vi "Shoot Teleop Handler.vi"(11 "Input Velocities":T1) -> ()   [LabVIEW 2025]
uses:
  swerve-template/Type Definitions/Data/Robot Velocities.ctl
  <vilib>/Rock Robotics/WPI/Joystick/XBox Buttons Indexer.ctl
  <vilib>/Rock Robotics/WPI/Joystick/XBox Axes Indexer.ctl
  Hopper/Implementation/Hopper Operations.ctl
  Transfer/Implementation/Transfer Operations.ctl
  Shooter/Implementation/Shooter Operations.ctl
  <vilib>/Rock Robotics/WPI/Utilities/WPI_GetSetVariantRefNum.vi
panel:
  in  "Steal Hood Setpoint":dbl=19.0
  in  "Steal Shot Velocity":dbl=8000.0
  in  "Hoard Hood Setpoint":dbl=19.0
  in  "Hoard Shot Velocity":dbl=4800.0
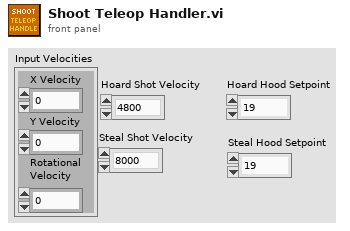
[diagram p1: front panel]
types:
  T1 = typedef "Robot Velocities.ctl" = cluster{"X Velocity":dbl, "Y Velocity":dbl, "Rotational \nVelocity":dbl}
  T2 = typedef "XBox Buttons Indexer.ctl" = enum16{"A", "B", "X", "Y", "Left Bumper", "Right Bumper", "Back", "Start", "Left Joystick", "Right Joystick"}
  T3 = typedef "XBox Axes Indexer.ctl" = enum16{"Left X", "Left Y", "Left Trigger", "Right Trigger", "Right X", "Right Y"}
  T4 = typedef "WPI_JoystickDevRef.ctl" = cluster{"Device":T5}
  T5 = typedef "WPI_JoystickDeviceEnum.ctl" = enum16{"USB 0", "USB 1", "USB 2", "USB 3", "USB 4", "USB 5"}
  T6 = typedef "Transfer Operations.ctl" = enum16{"Reserve", "Read Current", "Immediate", "Start Transfer"}
  T7 = typedef "Hopper Operations.ctl" = enum16{"Reserve", "Read Current", "Immediate", "Start Hopper"}
  T8 = typedef "Shooter Operations.ctl" = enum16{"Reserve", "Read Current", "Interpolated Shot", "Hood Manual", "Reset Hood", "Immediate", "Start Shooter"}
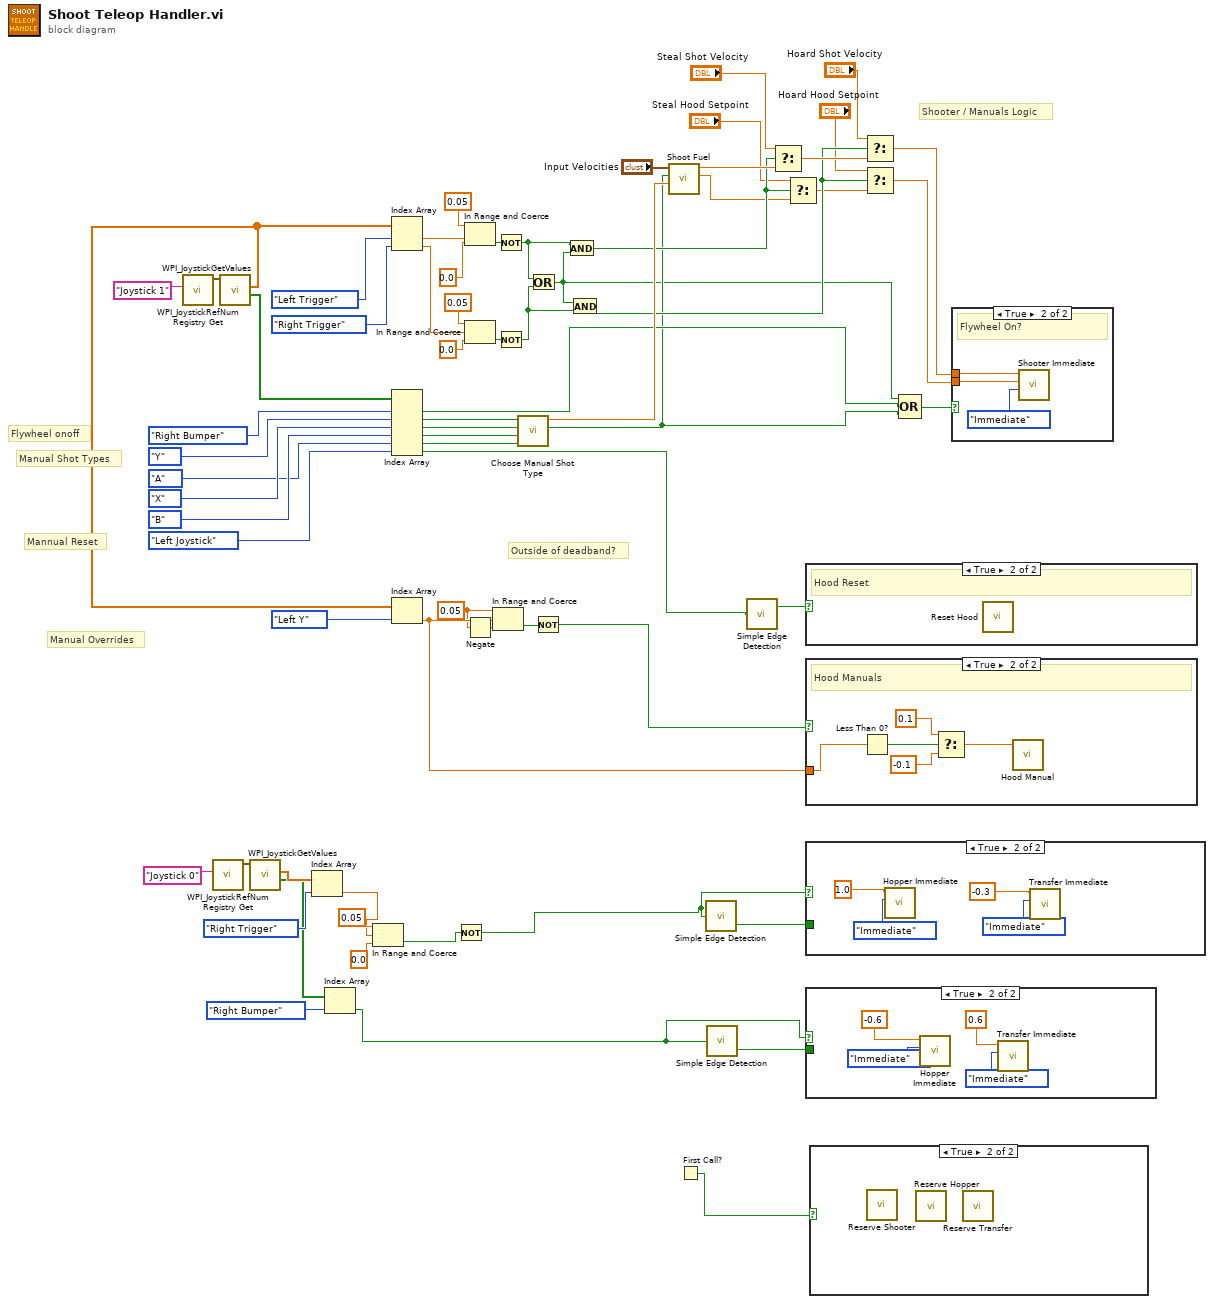
[diagram p0: block diagram]
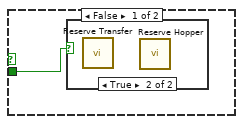
[diagram p3: hidden frame]
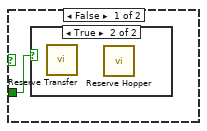
[diagram p6: hidden frame]
diagram:
  w49 = 0.05 ("upper limit")
  # "Outside of deadband?"
  # "Manual Overrides"
  # "Mannual Reset"
  # "Manual Shot Types"
  # "Flywheel onoff"
  # "Shooter / Manuals Logic"
  n1 = call <vilib>:"WPI_JoystickRefNum Registry Get.vi"("refnum name"="Joystick 1") -> ("JoystickDevRef"=w65:T4)  [unwired: 1 in, 9 out]
  n2 = call <vilib>:"WPI_JoystickRefNum Registry Get.vi"("refnum name"="Joystick 0") -> ("JoystickDevRef"=w52:T4)  [unwired: 1 in, 9 out]
  n3 = call <vilib>:"WPI_JoystickGetValues.vi"("JoystickDevRef"=w65) -> ("Buttons"=w64:bool[], "Axes"=w55:dbl[])  [unwired: 6 in, 3 out]
  n4 = call <vilib>:"WPI_JoystickGetValues.vi"("JoystickDevRef"=w52) -> ("Buttons"=w11:bool[], "Axes"=w16:dbl[])  [unwired: 6 in, 3 out]
  n5 = Index Array(array=w16, index=XBox_Axes_Indexer."Right Trigger" ("XBox Axes")) -> (element=w12:dbl)
  n6 = Index Array(array=w11, index=XBox_Buttons_Indexer."Right Bumper" ("XBox Buttons")) -> (element=w8:bool)
  n7 = In Range and Coerce(upper limit=0.05, x=w12, lower limit=0.0) -> (In Range?=w7:bool)  [unwired: 1 out]
  n8 = Index Array(array=w55, index #1=XBox_Axes_Indexer."Left Trigger" ("XBox Axes"), index #2=XBox_Axes_Indexer."Right Trigger" ("XBox Axes")) -> (element #1=w41:dbl, element #2=w38:dbl)
  n9 = Index Array(array=w64, index #1=XBox_Buttons_Indexer."Right Bumper" ("XBox Buttons"), index #2=XBox_Buttons_Indexer."Y" ("XBox Buttons"), index #3=XBox_Buttons_Indexer."X" ("XBox Buttons"), index #4=XBox_Buttons_Indexer."B" ("XBox Buttons"), index #5=XBox_Buttons_Indexer."A" ("XBox Buttons"), index #6=XBox_Buttons_Indexer."Left Joystick" ("XBox Buttons")) -> (element #1=w5:bool, element #2=w44:bool, element #3=w45:bool, element #4=w46:bool, element #5=w47:bool, element #6=w35:bool)
  n10 = Index Array(array=w55, index=XBox_Axes_Indexer."Left Y" ("XBox Axes")) -> (element=w51:dbl)
  n11 = Not(x=w7) -> (.not. x?=w6:bool)
  n12 = In Range and Coerce(upper limit=0.05, x=w41, lower limit=0.0) -> (In Range?=w36:bool)  [unwired: 1 out]
  n13 = In Range and Coerce(upper limit=0.05, x=w38, lower limit=0.0) -> (In Range?=w37:bool)  [unwired: 1 out]
  n14 = Negate(x=w49) -> (-x=w50:dbl)
  n15 = In Range and Coerce(upper limit=w49, x=w51, lower limit=w50) -> (In Range?=w48:bool)  [unwired: 1 out]
  n16 = Not(x=w36) -> (.not. x?=w30:bool)
  n17 = Not(x=w37) -> (.not. x?=w24:bool)
  n18 = call "Choose Manual Shot Type.vi"("1"=w47, "2"=w46, "3"=w45, "4"=w44) -> ("Manual Shot?"=w4:bool, "Manual Shot Distance"=w31:dbl)  [unwired: 6 in]
  n19 = Or(x=w30, y=w24) -> (x .or. y?=w3:bool)
  n20 = Not(x=w48) -> (.not. x?=w33:bool)
  n21 = And(x=w30, y=w3) -> (x .and. y?=w27:bool)
  n22 = And(x=w3, y=w24) -> (x .and. y?=w20:bool)
  n23 = call "Shoot Fuel.vi"("Manual Distance"=w31, "Manual Control?"=w4, "Input Velocities"="Input Velocities") -> ("Hood Setpoint"=w26:dbl, "Shooter RPM"=w29:dbl)  [unwired: 7 in]
  n24 = First Call?() -> (First Call?: T/F=w1:bool)
  n25 = call "Simple Edge Detection.vi"("In"=w6) -> ("Falling Edge"=w32:bool)  [unwired: 1 out]
  n26 = call "Simple Edge Detection.vi"("In"=w8) -> ("Falling Edge"=w9:bool)  [unwired: 1 out]
  n27 = call "Simple Edge Detection.vi"("In"=w35) -> ("Rising Edge"=w34:bool)  [unwired: 1 out]
  n28 = Select(t="Steal Shot Velocity", s=w27, f=w29) -> (s? t:f=w23:dbl)
  n29 = Select(t="Steal Hood Setpoint", s=w27, f=w26) -> (s? t:f=w19:dbl)
  n30 = case shown="True" w34 {
    frame False {
    }
    frame True {
      # "Hood Reset"
      n31 = call "Reset Hood.vi"() -> ()  [unwired: 11 in, 1 out]
    }
  }
  n32 = case shown="True" w33 {
    tunnel: w51 -> [_ w72]
    frame False {
      # "idek bru"
    }
    frame True {
      # "Hood Manuals"
      n33 = Less Than 0?(x=w72) -> (x < 0?=w71:bool)
      n34 = Select(t=0.1, s=w71, f=-0.1) -> (s? t:f=w68:dbl)
      n35 = call "Hood Manual.vi"("Setpoint"=w68) -> ()  [unwired: 10 in, 1 out]
    }
  }
  n36 = case shown="True" w6 {
    tunnel: w32 -> [w73 _]
    frame False {
      n37 = case shown="True" w73 {
        frame False {
        }
        frame True {
          n38 = call "Reserve Transfer.vi"() -> ()  [unwired: 11 in, 1 out]
          n39 = call "Reserve Hopper.vi"() -> ()  [unwired: 11 in, 1 out]
        }
      }
    }
    frame True {
      n40 = call "Hopper Immediate.vi"("Operation"=Hopper_Operations."Immediate", "Setpoint"=1.0) -> ()  [unwired: 9 in, 1 out]
      n41 = call "Transfer Immediate.vi"("Operation"=Transfer_Operations."Immediate", "Setpoint"=-0.3) -> ()  [unwired: 9 in, 1 out]
    }
  }
  n42 = case shown="True" w8 {
    tunnel: w9 -> [w78 _]
    frame False {
      n43 = case shown="True" w78 {
        frame False {
        }
        frame True {
          n44 = call "Reserve Transfer.vi"() -> ()  [unwired: 11 in, 1 out]
          n45 = call "Reserve Hopper.vi"() -> ()  [unwired: 11 in, 1 out]
        }
      }
    }
    frame True {
      n46 = call "Hopper Immediate.vi"("Operation"=Hopper_Operations."Immediate", "Setpoint"=-0.6) -> ()  [unwired: 9 in, 1 out]
      n47 = call "Transfer Immediate.vi"("Operation"=Transfer_Operations."Immediate", "Setpoint"=0.6) -> ()  [unwired: 9 in, 1 out]
    }
  }
  n48 = case shown="True" w1 {
    frame False {
    }
    frame True {
      n49 = call "Reserve Shooter.vi"() -> ()  [unwired: 11 in, 1 out]
      n50 = call "Reserve Hopper.vi"() -> ()  [unwired: 11 in, 1 out]
      n51 = call "Reserve Transfer.vi"() -> ()  [unwired: 11 in, 1 out]
    }
  }
  n52 = Select(t="Hoard Shot Velocity", s=w20, f=w23) -> (s? t:f=w22:dbl)
  n53 = Select(t="Hoard Hood Setpoint", s=w20, f=w19) -> (s? t:f=w17:dbl)
  n54 = Compound Arithmetic op=OR(w3, w5, w4) -> (w2:bool)
  n55 = case shown="True" w2 {
    tunnel: w22 -> [_ w85]
    tunnel: w17 -> [_ w84]
    frame False {
      # "Bumper not pressed..."
    }
    frame True {
      # "Flywheel On?"
      n56 = call "Shooter Immediate.vi"("Operation"=Shooter_Operations."Immediate", "Hood Setpoint"=w84, "Setpoint"=w85) -> ()  [unwired: 8 in, 1 out]
    }
  }
